vi "tearDown.vi"(8 "error in (no error)":errorcluster, 11 "reference in":refnum<class "Bus Controller Suite.lvclass">) -> (0 "error out":errorcluster, 3 "reference out":refnum<class "Bus Controller Suite.lvclass">)   [LabVIEW 2016, in "Bus Controller Suite.lvclass"]
doc: "tearDown runs after the test method has completed. Use this method to clean up any operations or references that were opened by setUp or the test method. Unit tests should be independent of other unit tests so this VI should ensure that the next test can run in a 'clean' test environment."
uses:
  Bus Controller Suite.lvclass
  Utilities/Simulated FPGA/FPGA Sim.lvclass
  Bus Controller Suite.lvclass/Bus Controller Suite.ctl
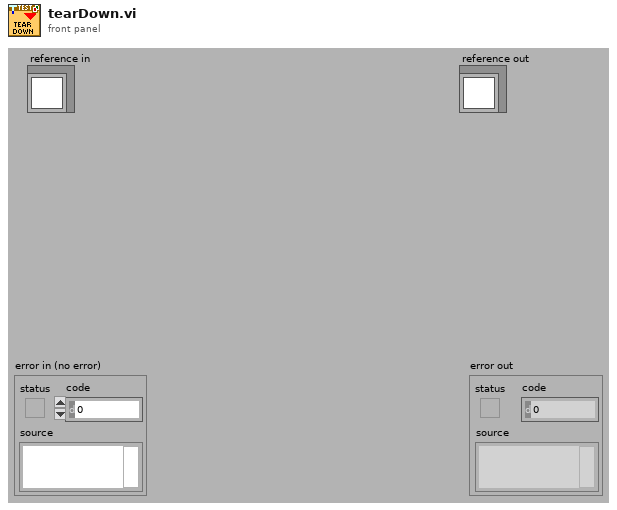
[diagram p1: front panel]
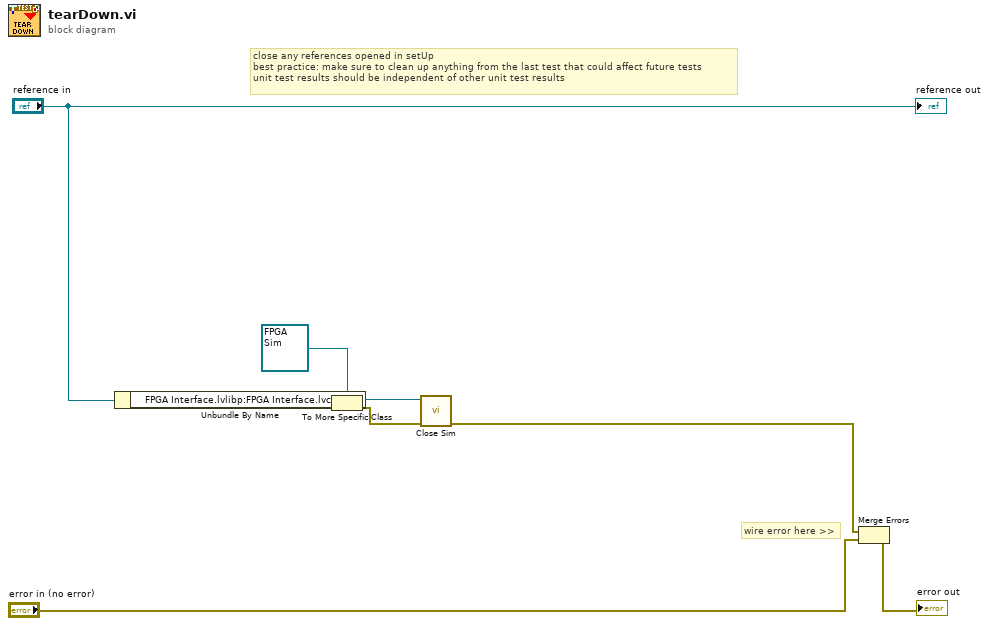
[diagram p0: block diagram]
diagram:
  # "wire error here >>"
  # "close any references opened in setUp\nbest practice: make sure to clean up anything from the last test that could affect future tests\nunit test results should be independent of other unit test results"
  n1 = Unbundle By Name("reference in") -> ("FPGA Interface.lvlibp:FPGA Interface.lvclass"=w6:refnum<class "FPGA Interface.lvclass">)
  n2 = To More Specific Class(target class=refnum<class "FPGA Sim.lvclass"> refnum ("FPGA Sim.lvclass"), reference=w6) -> (specific class reference=w5:refnum<class "FPGA Sim.lvclass">, error out=w2:errorcluster)  [unwired: 1 in]
  n3 = call "Close Sim.vi"("error in (no error)"=w2, "FPGA Sim in"=w5) -> ("error out"=w1:errorcluster)  [unwired: 9 in]
  n4 = Merge Errors(w1, "error in (no error)") -> (→"error out":errorcluster)
  "reference out" <- "reference in"
